vi "Shutdown.vi"(8 "error in (no error)":errorcluster, 11 "Force Test Stand in":refnum<class "Force Test Stand.lvclass">) -> (0 "error out":errorcluster, 3 "Force Test Stand out":refnum<class "Force Test Stand.lvclass">)   [LabVIEW 2018, in "Force Test Stand.lvlib" / "Force Test Stand.lvclass"]
uses:
  Force Test Stand.lvclass
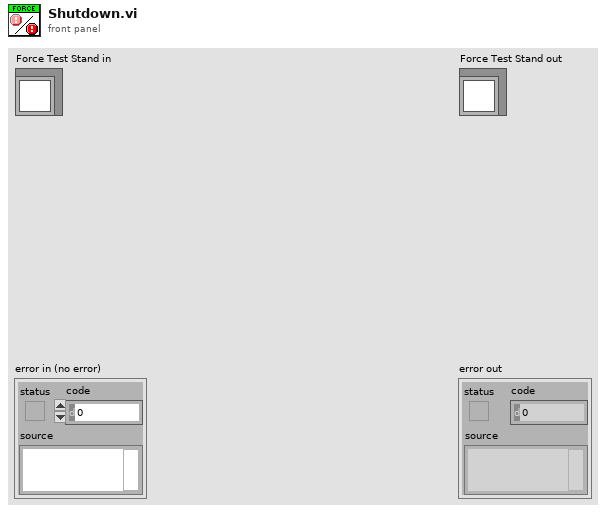
[diagram p1: front panel]
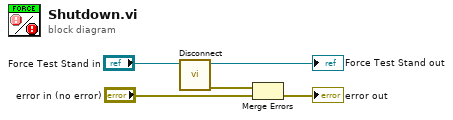
[diagram p0: block diagram]
diagram:
  n1 = call-dynamic "Disconnect.vi"("Force Test Stand in"="Force Test Stand in") -> ("error out"=w5:errorcluster, "Force Test Stand out"=→"Force Test Stand out":refnum<class "Force Test Stand.lvclass">)  [unwired: 9 in]
  n2 = Merge Errors(w5, "error in (no error)") -> (→"error out":errorcluster)
